vi "Set Splitter.vi"(8 "error in (no error)":errorcluster, 9 "Splitter Reference":refnum<vi>, 10 "Splitter Name":string, 11 "IViewManager in":refnum<class "IViewManager.lvclass">) -> (0 "error out":errorcluster, 3 "IViewManager out":refnum<class "IViewManager.lvclass">)   [LabVIEW 2017, in "IViewManager.lvlib" / "IViewManager.lvclass"]
uses:
  <vilib>/gpm_packages/@cs/mva-viewable/Source/IViewManager/IViewManager/IViewManager.lvclass
  <vilib>/gpm_packages/@cs/mva-viewable/Source/IViewManager/IViewManager/IViewManager.lvclass/IViewManager.ctl
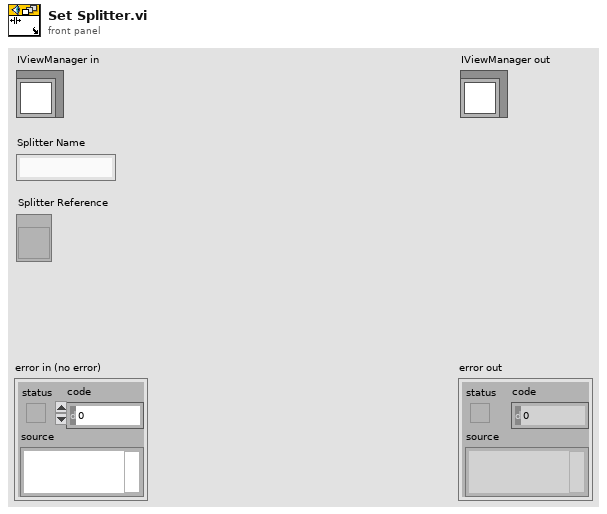
[diagram p1: front panel]
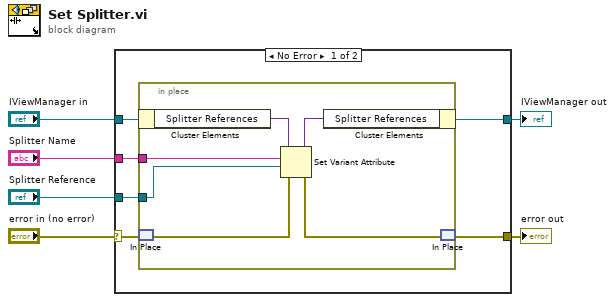
[diagram p0: block diagram]
diagram:
  n1 = case shown="No Error" "error in (no error)" {
    selector: "error in (no error)" -> [w9 w20]
    tunnel: "IViewManager in" -> [w12 w19]
    tunnel: [w7 w19] -> w1
    tunnel: "Splitter Name" -> [w11 _]
    tunnel: "Splitter Reference" -> [w10 _]
    tunnel: [w8 w20] -> w2
    frame No Error {
      n2 = in-place {
        in-place-border: w11 -> [w18]
        in-place-border: w10 -> [w16]
        n3 = in-place-cluster #1(w12) -> ("Splitter References"=w13:variant)
        n4 = in-place-match #2(w9) -> (w15:errorcluster)
        n5 = Set Variant Attribute(Variant=w13, name=w18, value=w16, error in=w15) -> (Variant out=w17:variant, error out=w14:errorcluster)  [unwired: 1 out]
        n6 = in-place-cluster #1("Splitter References"=w17) -> (w7:refnum<class "IViewManager.lvclass">)
        n7 = in-place-match #2(w14) -> (w8:errorcluster)
      }
    }
    frame Error {
    }
  }
  "error out" <- w2
  "IViewManager out" <- w1
